vi "Read L2 Enet FIFO.vi"(8 "error in (no error)":errorcluster, 9 "Timeout (ms)":i32, 10 "Data in":u8[](array[numeric]), 11 "CIF_Fifo_L2Enet_Multi in":refnum<class "CIF_Fifo_L2Enet_Multi.lvclass">) -> (0 "error out":errorcluster, 1 "timed out?":bool, 2 "Data out":u8[](array[numeric]), 3 "CIF_Fifo_L2Enet_Multi out":refnum<class "CIF_Fifo_L2Enet_Multi.lvclass">, 4 "Header":T1)   [LabVIEW 2021, in "CIF_Fifo_L2Enet_Multi.lvclass"]
uses:
  CIF_Fifo_L2Enet_Multi.lvclass
  ChannelCommon/typedef/FIFO Header.ctl
  CIF_Fifo_L2Enet_Multi.lvclass/CIF_Fifo_L2Enet_Multi.ctl
  ChannelCommon/ChannelCommon.lvlib
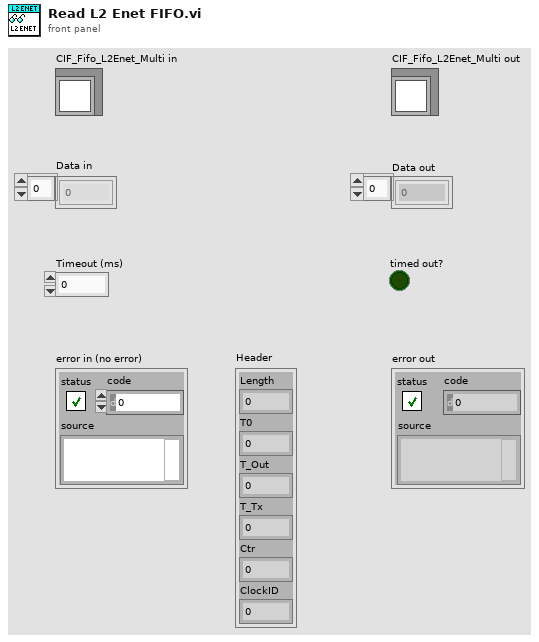
[diagram p1: front panel]
types:
  T1 = typedef "ChannelCommon.lvlib/FIFO Header.ctl" = cluster{"Length":u64, "T0":i64, "T_Out":i64, "T_Tx":i64, "Ctr":u64, "ClockID":u8}
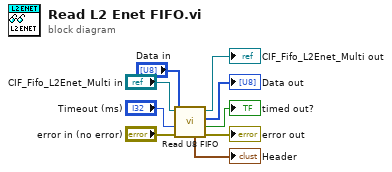
[diagram p0: block diagram]
diagram:
  n1 = call-dynamic "Read U8 FIFO.vi"("error in (no error)"="error in (no error)", "Timeout (ms)"="Timeout (ms)", "Data in"="Data in", "CIFFIFO in"="CIF_Fifo_L2Enet_Multi in") -> ("error out"=→"error out":errorcluster, "timed out?"=→"timed out?":bool, "Data out"=→"Data out":u8[], "CIFFIFO out"=→"CIF_Fifo_L2Enet_Multi out":refnum<class "CIF_Fifo_L2Enet_Multi.lvclass">, "Header"=→"Header":T1)  [unwired: 3 in]
